vi "Get Measured Flow Rate.vi"(8 "error in (no error)":errorcluster, 11 "RRG in":refnum<class "Eltochpribor RRG.lvclass">) -> (0 "error out":errorcluster, 2 "measured flow rate, %":dbl, 3 "RRG out":refnum<class "Eltochpribor RRG.lvclass">)   [LabVIEW 2015, in "Eltochpribor RRG.lvclass"]
doc: "Gets measured flow rate as a percentage of full scale calibrated flow rate."
uses:
  Eltochpribor RRG.lvclass
  Modbus Client/PL Modbus Client.lvclass
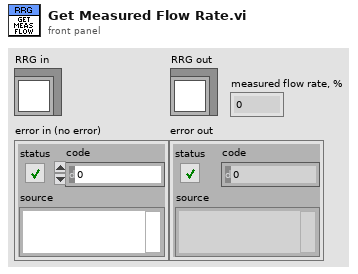
[diagram p1: front panel]
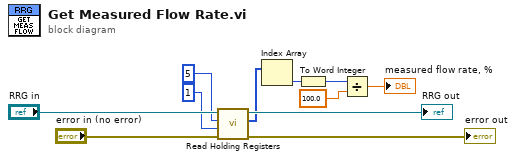
[diagram p0: block diagram]
diagram:
  n1 = call "Read Holding Registers.vi"("error in (no error)"="error in (no error)", "number of holding registers"=u16 1, "address"=u16 5, "MODBUS in"="RRG in") -> ("error out"=→"error out":errorcluster, "values"=w5:u16[], "MODBUS out"=→"RRG out":refnum<class "Eltochpribor RRG.lvclass">)  [unwired: 5 in]
  n2 = Index Array(array=w5) -> (element=w4:u16)  [unwired: 1 in]
  n3 = To Word Integer(number=w4) -> (16bit integer=w1:i16)
  n4 = Divide(x=w1, y=100.0) -> (x/y=→"measured flow rate, %":dbl)
